vi "Read Name.vi"(8 "error in (no error)":errorcluster, 11 "Order Item in":refnum<class "Order Item.lvclass">) -> (0 "error out":errorcluster, 2 "Name":string, 3 "Order Item out":refnum<class "Order Item.lvclass">)   [LabVIEW 2020, in "Order Item.lvclass"]
doc: "Read Name accessor VI"
uses:
  Order Item.lvclass
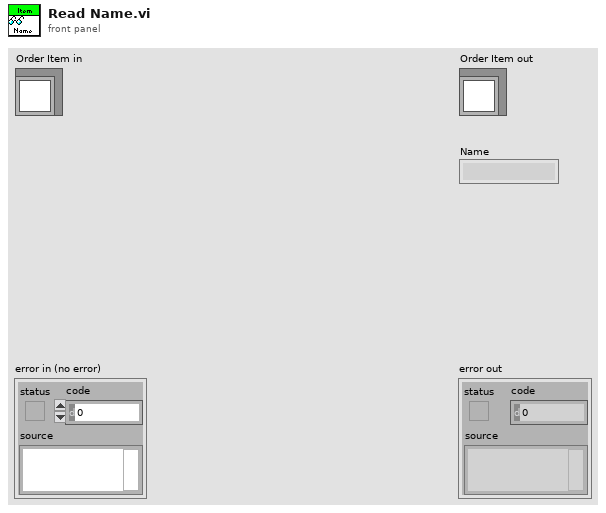
[diagram p1: front panel]
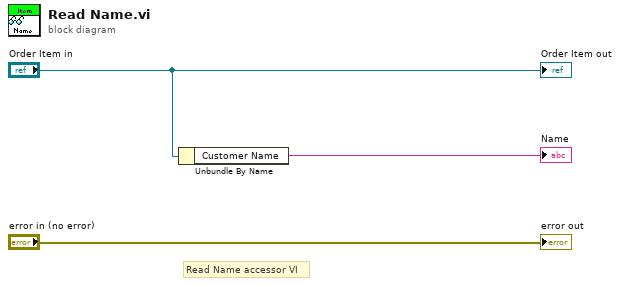
[diagram p0: block diagram]
diagram:
  # "Read Name accessor VI"
  n1 = Unbundle By Name("Order Item in") -> ("Customer Name"=→"Name":string)
  "error out" <- "error in (no error)"
  "Order Item out" <- "Order Item in"
